vi "Spark MAX Write Parameter Cache.vi"(8 "error in (no error)":errorcluster, 9 "string":string, 10 "Variant":variant, 11 "Data Value Reference in":refnum<data-value>) -> (0 "error out":errorcluster)   [LabVIEW 2019]
panel:
  # "Use non-reentrant VI to force synchronization"
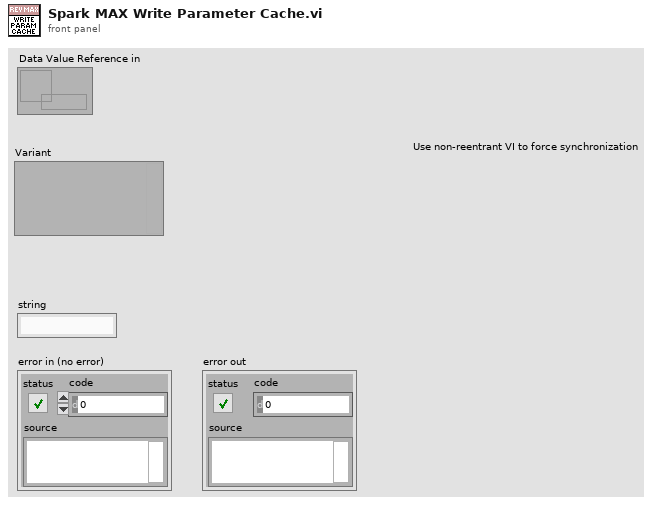
[diagram p1: front panel]
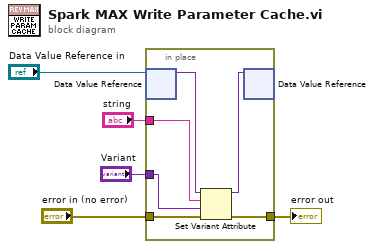
[diagram p0: block diagram]
diagram:
  n1 = in-place {
    in-place-border: "error in (no error)" -> [w11]
    in-place-border: [w10] -> w3
    in-place-border: "string" -> [w9]
    in-place-border: "Variant" -> [w6]
    n2 = in-place-dvr #1("Data Value Reference in") -> (w8:variant)  [unwired: 1 out]
    n3 = Set Variant Attribute(Variant=w8, name=w9, value=w6, error in=w11) -> (Variant out=w7:variant, error out=w10:errorcluster)  [unwired: 1 out]
    n4 = in-place-dvr #1(w7) -> ()  [unwired: 2 out]
  }
  "error out" <- w3
